vi "subFD_FXP CodeGen.vi"() -> ()   [LabVIEW 2023]
uses:
  <vilib>/addons/Digital Filter Design/_Objects.llb/DFD Filter Obj.ctl
  <vilib>/addons/Digital Filter Design/_Objects.llb/DFD Filter Coef.ctl
  <vilib>/addons/Digital Filter Design/_Objects.llb/DFD Filter Structure Type Selector.ctl
  <vilib>/addons/Digital Filter Design/_Objects.llb/dfd_Internal Quantization Settings.ctl
  <vilib>/addons/Digital Filter Design/_Objects.llb/dfd_Internal Quantization Srcs.ctl
  <vilib>/addons/Digital Filter Design/_Objects.llb/DFD Coef Norm Type.ctl
  <vilib>/Utility/error.llb/ErrWarn.ctl
  <vilib>/Utility/cursorutil.llb/Set Cursor (Icon Pict).vi
  <vilib>/addons/Digital Filter Design/CodeGen.llb/DFD FXP C Code Generator.vi
  <vilib>/addons/Digital Filter Design/CodeGen.llb/DFD FXP Integer LabVIEW Code Generator.vi
  <vilib>/addons/Digital Filter Design/CodeGen.llb/DFD FXP LabVIEW FPGA Code Generator.vi
  <vilib>/addons/Digital Filter Design/NI_DigFilterLicensed.lvlib
panel:
  out "error":T1=TRUE
  out "Maximum Input Fs@40 MHz FPGA Clock":string
  out "Message":string="Code that engineers commonly use to program target DSP hardware. You can directly compile the generated code to run on a fixed-point DSP."
  in  "# Channels":i32=1
  in  "Filter Name":string="MyFilter"
  in  "Destination Folder":path
  out "Code Example":u16(ring)
  in  "Code Type":enum32{"C", "integer LV", "SCTL LV"}(radio)
  out "Successful Design?":bool
  out "filter out":T2={"mSRate_Fs"=1.0, "mSRate_Version"="1.0", "mSRate_Comments"="", "mSRate_OrgCoef"={"type"=enum."Undefined", "gain"=1.0, "coef a (k)"=[], "coef b (v)"=[]}, "mSRate_CurCoef"={"type"=enum."Undefined", "gain"=1.0, "coef a (k)"=[], "coef b (v)"=[]}, "mSRate_Quantized?"=FALSE, "mSRate_QCoef"={"type"=enum."Undefined", "gain"=1.0, "coef a (k)"=[], "coef b (v)"=[]}, "mSRate_QSettings"=[], "mSRate_Order"=0, "mSRate_Scaling"={"mSRate_ScaleByPowerOf2?"=FALSE, "mSRate_ScaleType"=enum."No Norm"}} {"mSRate_QSettings"."source" items=["Coef a/k"=0, "Coef b/v"=7, "Input"=1, "Output"=2, "Multiplicand"=3, "Product"=4, "Sum"=5, "Delay"=6, "Gain"=8]}
  in  "filter in":T2={"mSRate_Fs"=1.0, "mSRate_Version"="1.0", "mSRate_Comments"="", "mSRate_OrgCoef"={"type"=enum."Undefined", "gain"=1.0, "coef a (k)"=[], "coef b (v)"=[]}, "mSRate_CurCoef"={"type"=enum."Undefined", "gain"=1.0, "coef a (k)"=[], "coef b (v)"=[]}, "mSRate_Quantized?"=FALSE, "mSRate_QCoef"={"type"=enum."Undefined", "gain"=1.0, "coef a (k)"=[], "coef b (v)"=[]}, "mSRate_QSettings"=[], "mSRate_Order"=0, "mSRate_Scaling"={"mSRate_ScaleByPowerOf2?"=FALSE, "mSRate_ScaleType"=enum."No Norm"}} {"mSRate_QSettings"."source" items=["Coef a/k"=0, "Coef b/v"=7, "Input"=1, "Output"=2, "Multiplicand"=3, "Product"=4, "Sum"=5, "Delay"=6, "Gain"=8]}
  in  "Generate Code":bool
  out "OK":bool
  in  "stop":bool
  # "Code Example"
  # "Code Type"
  # "Options"
  # "Code Generation Settings"
  # "Code Generation Feedback"
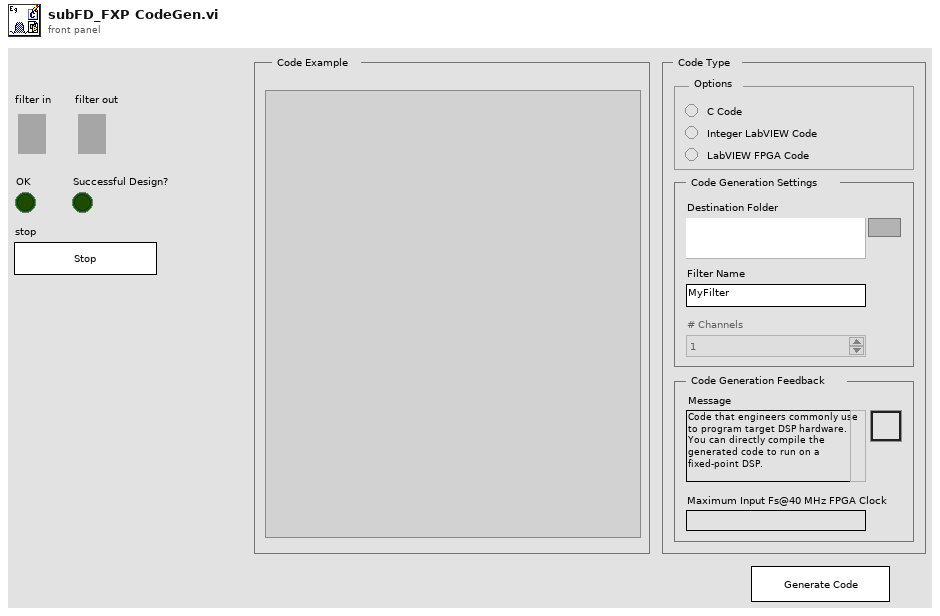
[diagram p1: front panel]
types:
  T1 = typedef "ErrWarn.ctl" = bool
  T2 = typedef "NI_DigFilterLicensed.lvlib/DFD Filter Obj.ctl" = cluster{"mSRate_Fs":dbl, "mSRate_Version":string, "mSRate_Comments":string, "mSRate_OrgCoef":T3, "mSRate_CurCoef":T3, "mSRate_Quantized?":bool, "mSRate_QCoef":T3, "mSRate_QSettings":T5[], "mSRate_Order":i32, "mSRate_Scaling":cluster{"mSRate_ScaleByPowerOf2?":bool, "mSRate_ScaleType":T7}}
  T3 = typedef "NI_DigFilterLicensed.lvlib/DFD Filter Coef.ctl" = cluster{"type":T4, "gain":dbl, "coef a (k)":dbl[], "coef b (v)":dbl[]}
  T4 = typedef "NI_DigFilterLicensed.lvlib/DFD Filter Structure Type Selector.ctl" = enum16{"Undefined", "FIR Direct Form", "FIR Direct Form Transposed", "FIR Symmetric", "FIR Antisymmetric", "IIR Direct Form I", "IIR Direct Form I Transposed", "IIR Direct Form II", "IIR Direct Form II Transposed", "IIR Cascaded Second Order Sections Form I", "IIR Cascaded Second Order Sections Form I Transposed", "IIR Cascaded Second Order Sections Form II", "IIR Cascaded Second Order Sections Form II Transposed", "Lattice Allpass (basic sections)", "Lattice Allpass (one multiplier sections)", "Lattice Allpass (normalized sections)", "Lattice AR (basic sections)", "Lattice AR (one multiplier sections)", "Lattice AR (normalized sections)", "Lattice MA (minimum phase)", "Lattice MA (maximum phase)", "Lattice ARMA (basic sections)", "Lattice ARMA (one multiplier sections)", "Lattice ARMA (normalized sections)"}
  T5 = typedef "NI_DigFilterLicensed.lvlib/dfd_Internal Quantization Settings.ctl" = cluster{"source":T6, "wl":i16, "iwl":i16, "overflow mode":enum16{"Saturation", "Wrap"}, "rounding mode":enum16{"Nearest", "Truncation"}, "signed?":bool}
  T6 = typedef "NI_DigFilterLicensed.lvlib/dfd_Internal Quantization Srcs.ctl" = u16
  T7 = typedef "NI_DigFilterLicensed.lvlib/DFD Coef Norm Type.ctl" = enum16{"No Norm", "Time Domain 1-Norm", "Time Domain 2-Norm", "Time Domain Inf-Norm"}
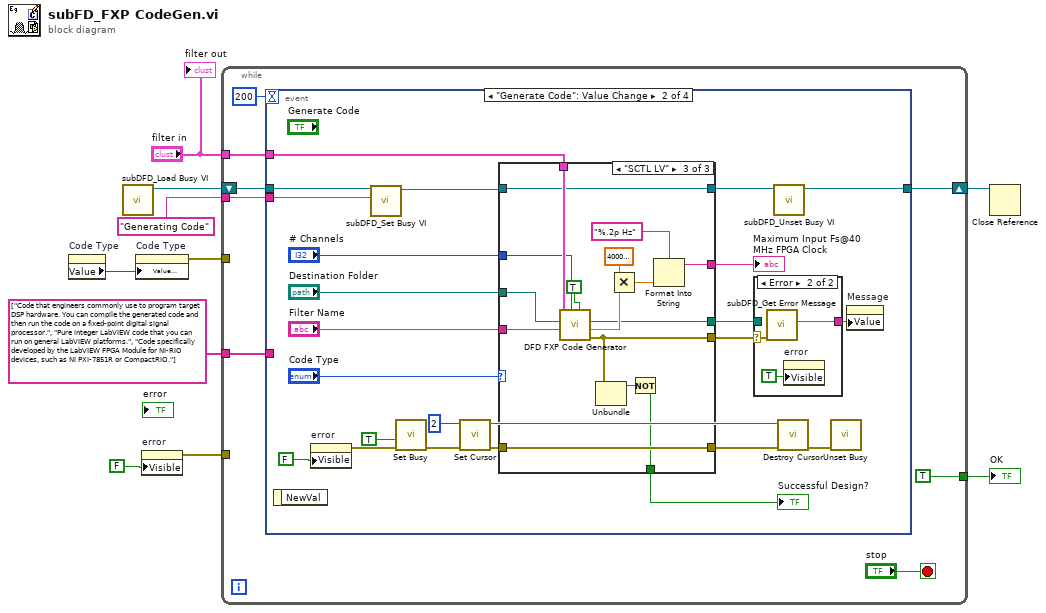
[diagram p0: block diagram]
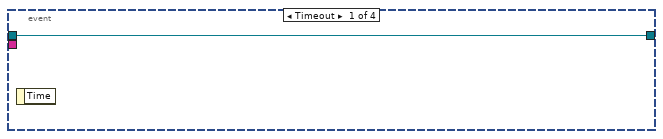
[diagram p2: hidden frame]
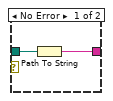
[diagram p3: hidden frame]
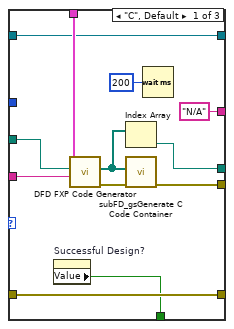
[diagram p4: hidden frame]
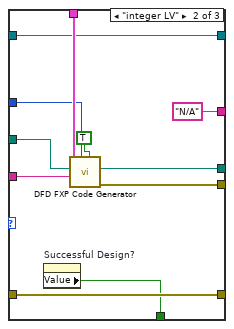
[diagram p5: hidden frame]
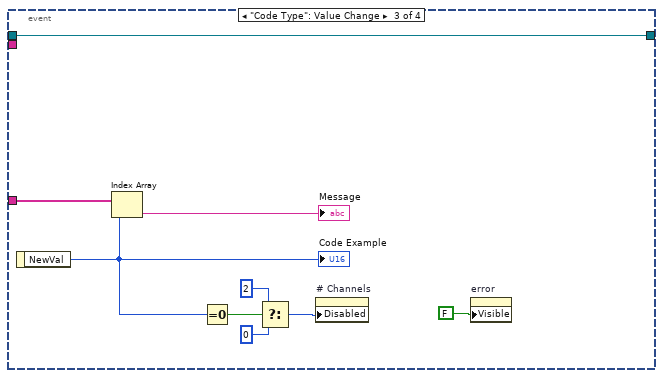
[diagram p6: hidden frame]
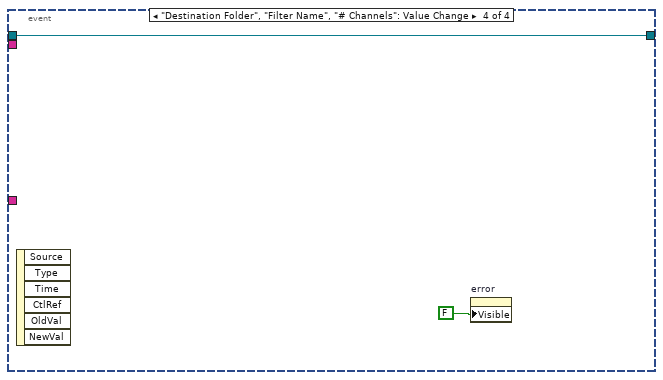
[diagram p7: hidden frame]
diagram:
  n1 = property on="Code Type" class="RadioBtnsControl (strict)"() -> ("Value"=w8:enum32{"C", "integer LV", "SCTL LV"})  [unwired: 2 in, 2 out]
  n2 = call <vilib>:"subDFD_Load Busy VI.vi"() -> ("Busy vi reference"=w2:refnum<vi>)  [unwired: 11 out]
  n3 = property on="Code Type" class="RadioBtnsControl (strict)"("Value (Signaling)"=w8) -> (error out=w7:errorcluster)  [unwired: 2 in, 1 out]
  n4 = property on="error" class="Bool"("Visible"=FALSE) -> (error out=w3:errorcluster)  [unwired: 2 in, 1 out]
  n5 = while {
    tunnel: [TRUE] -> w10
    tunnel: string[] ["Code that engineers commonly use to program target DSP hardware. You can compile the generated code and then run the code on a fixed-point digital signal processor.", "Pure integer LabVIEW code that you can run on general LabVIEW platforms.", "Code specifically developed by the LabVIEW FPGA Module for NI-RIO devices, such as NI PXI-7851R or CompactRIO."] -> [w15]
    tunnel: w7 -> [_]
    tunnel: "filter in" -> [w14]
    shift-right: [w12] -> w5
    shift-left: w2 -> [w13]
    tunnel: w3 -> [_]
    tunnel: "Generating Code" ("control name") -> [w11]
    stop <- "stop" stop-if-true
    n6 = event shown="[1] \"Generate Code\": Value Change" {
      selector: _ -> [_ _ _ _]
      dyn-events: _ -> [_ _ _ _]
      timeout: 200 -> [_ _ _ _]
      tunnel: w15 -> [_ _ w96 _]
      tunnel: w14 -> [_ w42 _ _]
      tunnel: w13 -> [w19 w26 w89 w98]
      tunnel: [w19 w27 w89 w98] -> w12
      tunnel: w11 -> [_ w20 _ _]
      event Timeout {
        n7 = event-data() -> ()  [unwired: 2 out]
      }
      event "Generate Code": Value Change {
        n8 = event-data() -> ()  [unwired: 2 out]
        n9 = property on="error" class="Bool"("Visible"=FALSE) -> (error out=w21:errorcluster)  [unwired: 2 in, 1 out]
        n10 = call <vilib>:"subDFD_Set Busy VI.vi"("busy task"=w20, "Busy vi reference"=w26) -> ("dup Busy vi reference"=w25:refnum<vi>)  [unwired: 1 in, 8 out]
        n11 = call <vilib>:"Set Busy.vi"("error in (no error)"=w21, "disable click? (T)"=TRUE) -> ("error out"=w40:errorcluster)  [unwired: 2 in, 7 out]
        n12 = call-poly <vilib>:"Set Cursor.vi"("error in (no error)"=w40, "icon"=u16 2) -> ("error out"=w39:errorcluster, "previous cursor ID"=w35:refnum<k1>)  [unwired: 1 in, 7 out]
        n13 = case shown="\"SCTL LV\"" "Code Type" {
          tunnel: w42 -> [w60 w71 w87]
          tunnel: [w58 w69 w77] -> w30
          tunnel: w39 -> [w57 w68 w85]
          tunnel: [w57 w68 w85] -> w37
          tunnel: [w56 w67 w75] -> w34
          tunnel: "Filter Name" -> [w53 w63 w80]
          tunnel: "Destination Folder" -> [w55 w65 w83]
          tunnel: "# Channels" -> [_ w66 w84]
          tunnel: ["N/A" "N/A" w72] -> w29
          tunnel: w25 -> [w52 w62 w79]
          tunnel: [w52 w62 w79] -> w28
          tunnel: [w49 w61 w78] -> w23
          frame "C", Default {
            n14 = property on="Successful Design?" class="Bool (strict)"() -> ("Value"=w56:bool)  [unwired: 2 in, 2 out]
            n15 = call-poly <vilib>:"DFD FXP Code Generator.vi"("filter name"=w53, "destination folder"=w55, "filter in"=w60) -> ("error out"=w59:errorcluster, "output files"=w50:path[])  [unwired: 2 in, 5 out]
            n16 = Index Array(array=w50) -> (element=w49:path)  [unwired: 1 in]
            n17 = call "subFD_gsGenerate C Code Container.vi"("error in (no error)"=w59, "output files"=w50) -> ("error out"=w58:errorcluster)  [unwired: 9 out]
            n18 = Wait (ms)(milliseconds to wait=u32 200) -> ()  [unwired: 1 out]
          }
          frame "integer LV" {
            n19 = property on="Successful Design?" class="Bool (strict)"() -> ("Value"=w67:bool)  [unwired: 2 in, 2 out]
            n20 = call-poly <vilib>:"DFD FXP Code Generator.vi"("open project? (F)"=TRUE ("open FP? (F)"), "# channels"=w66, "filter name"=w63, "destination folder"=w65, "filter in"=w71) -> ("error out"=w69:errorcluster, "lvproj path"=w61:path)  [unwired: 2 in, 3 out]
          }
          frame "SCTL LV" {
            n21 = call-poly <vilib>:"DFD FXP Code Generator.vi"("open project? (F)"=TRUE ("open FP? (F)"), "# channels"=w84, "filter name"=w80, "destination folder"=w83, "filter in"=w87) -> ("error out"=w77:errorcluster, "sampling frequency/FPGA clock"=w82:dbl, "lvproj path"=w78:path)  [unwired: 2 in, 2 out]
            n22 = Unbundle(w77) -> ("status"=w76:bool)  [unwired: 2 out]
            n23 = Multiply(x=40000000.0, y=w82) -> (x*y=w73:dbl)
            n24 = Not(x=w76) -> (.not. x?=w75:bool)
            n25 = Format Into String(format string="%.2p Hz", w73) -> (resulting string=w72:string)  [unwired: 2 in, 1 out]
          }
        }
        "Successful Design?" <- w34
        "Maximum Input Fs@40 MHz FPGA Clock" <- w29
        n26 = case shown="Error" w30 {
          selector: w30 -> [_ w48]
          tunnel: [w44 w47] -> w24
          tunnel: w23 -> [w45 _]
          frame No Error {
            n27 = Path To String(path=w45) -> (string=w44:string)
          }
          frame Error {
            n28 = call <vilib>:"subDFD_Get Error Message.vi"("error in (no error)"=w48) -> ("Error Message"=w47:string)  [unwired: 10 out]
            n29 = property on="error" class="Bool"("Visible"=TRUE) -> ()  [unwired: 2 in, 2 out]
          }
        }
        n30 = call <vilib>:"subDFD_Unset Busy VI.vi"("Busy vi reference"=w28) -> ("dup Busy vi reference"=w27:refnum<vi>)  [unwired: 1 in, 9 out]
        n31 = call <vilib>:"Destroy Cursor.vi"("cursor ID"=w35, "error in (no error)"=w37) -> ("error out"=w36:errorcluster)  [unwired: 8 out]
        n32 = call <vilib>:"Unset Busy.vi"("error in (no error)"=w36) -> ()  [unwired: 1 in, 10 out]
        n33 = property on="Message" class="Str"("Value"=w24) -> ()  [unwired: 2 in, 2 out]
      }
      event "Code Type": Value Change {
        n34 = event-data() -> ("NewVal"=w94:enum32{"C", "integer LV", "SCTL LV"})  [unwired: 1 out]
        "Code Example" <- w94
        n35 = Index Array(array=w96, index=w94) -> (element=→"Message":string)
        n36 = Equal To 0?(x=w94) -> (x = 0?=w93:bool)
        n37 = Select(t=u8 2 ("Disabled"), s=w93, f=u8 0) -> (s? t:f=w90:u8)
        n38 = property on="# Channels" class="DigNum (strict)"("Disabled"=w90) -> ()  [unwired: 2 in, 2 out]
        n39 = property on="error" class="Bool"("Visible"=FALSE) -> ()  [unwired: 2 in, 2 out]
      }
      event "Destination Folder", "Filter Name", "# Channels": Value Change {
        n40 = event-data() -> ()  [unwired: 7 out]
        n41 = property on="error" class="Bool"("Visible"=FALSE) -> ()  [unwired: 2 in, 2 out]
      }
    }
  }
  "OK" <- w10
  n42 = Close Reference(reference=w5) -> ()  [unwired: 1 in, 1 out]
  "filter out" <- "filter in"
